vi "Correct ID.vi"(11 "id in":string) -> (3 "corrected id out":string)   [LabVIEW 2020, in "Configuration_Helper.lvlib"]
uses:
  Configuration_Helper.lvlib
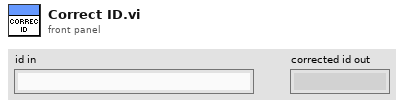
[diagram p1: front panel]
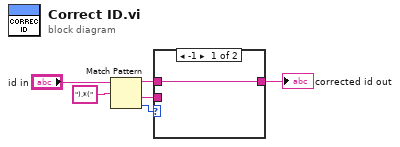
[diagram p0: block diagram]
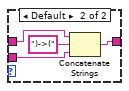
[diagram p2: hidden frame]
diagram:
  n1 = Match Pattern(string="id in", regular expression=").*(") -> (before substring=w4:string, after substring=w3:string, offset past match=w1:i32)  [unwired: 1 in, 1 out]
  n2 = case shown="-1" w1 {
    tunnel: w4 -> [w7 w11]
    tunnel: w3 -> [_ w10]
    tunnel: [w7 w8] -> w2
    frame -1 {
    }
    frame Default {
      n3 = Concatenate Strings(w11, ")->(" ("string"), w10) -> (w8:string)
    }
  }
  "corrected id out" <- w2
